vi "Example - Open Close CCD.vi"(8 "error in (no error)":errorcluster, 11 "CCD in":refnum<class "CCD.lvclass">) -> (0 "error out":errorcluster, 2 "device is open?":bool, 3 "CCD out":refnum<class "CCD.lvclass">)   [LabVIEW 2023, in "CCD.lvclass"]
uses:
  CCD.lvclass
  CCD.lvclass/CCD.ctl
panel:
  # "Connector Pane"
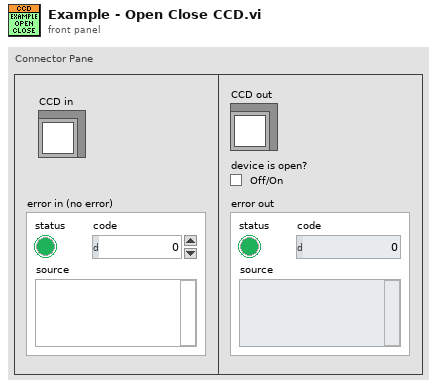
[diagram p1: front panel]
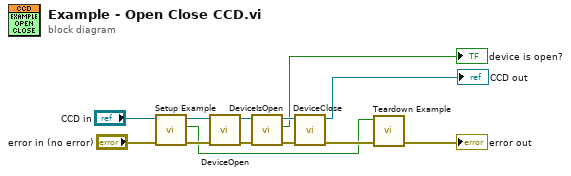
[diagram p0: block diagram]
diagram:
  n1 = call "Setup Example.vi"("error in (no error)"="error in (no error)", "CCD in"="CCD in") -> ("error out"=w7:errorcluster, "Module Was Already Running?"=w1:bool, "CCD out"=w3:refnum<class "CCD.lvclass">)  [unwired: 7 in]
  n2 = call-dynamic "DeviceOpen.vi"("error in (no error)"=w7, "CCD in"=w3) -> ("error out"=w13:errorcluster, "CCD out"=w9:refnum<class "CCD.lvclass">)  [unwired: 6 in, 2 out]
  n3 = call-dynamic "DeviceIsOpen.vi"("error in (no error)"=w13, "CCD in"=w9) -> ("error out"=w12:errorcluster, "device is open?"=→"device is open?":bool, "CCD out"=w10:refnum<class "CCD.lvclass">)  [unwired: 6 in, 1 out]
  n4 = call-dynamic "DeviceClose.vi"("error in (no error)"=w12, "CCD in"=w10) -> ("error out"=w4:errorcluster, "CCD out"=→"CCD out":refnum<class "CCD.lvclass">)  [unwired: 5 in, 3 out]
  n5 = call "Teardown Example.vi"("error in (no error)"=w4, "Module Was Already Running?"=w1) -> ("error out"=→"error out":errorcluster)  [unwired: 9 in]
